vi "Measurement API.vi"(7 "Action":T1, 8 "error IO":errorcluster) -> (0 "error IO 2":errorcluster, 2 "Temps":dbl[](array[numeric]))   [LabVIEW 2019]
uses:
  <vilib>/ULx/Create Channel.llb/ULx Create Channel (AI-Temperature).vi
  <vilib>/Utility/error.llb/DialogType.ctl
  <vilib>/ULx/Read.llb/ULx Read (Analog 1D DBL NChan 1Samp).vi
  <vilib>/Utility/file.llb/Read From Spreadsheet File (DBL).vi
  Measurement Action.ctl
panel:
  out "Mtr Brg Offsets":dbl[](array[numeric]) format="%0.3f"
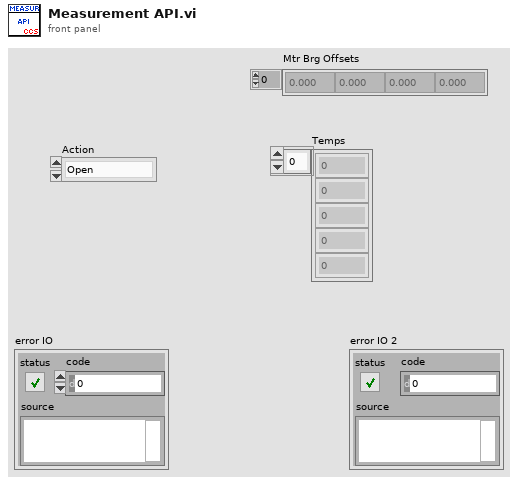
[diagram p1: front panel]
types:
  T1 = typedef "Measurement Action.ctl" = enum16{"Open", "Read Bearing Temps", "Read Motor Temps", "Close"}
  T2 = typedef "DialogType.ctl" = u16
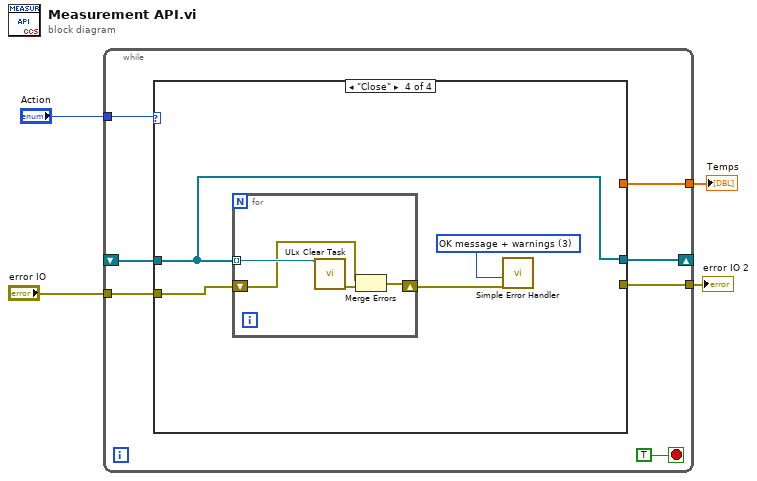
[diagram p0: block diagram]
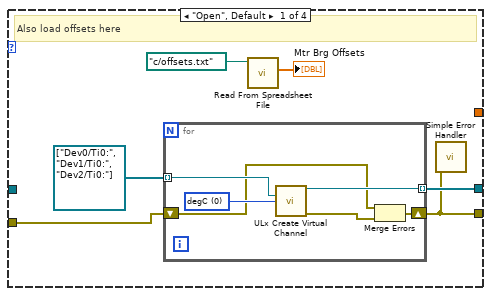
[diagram p2: hidden frame]
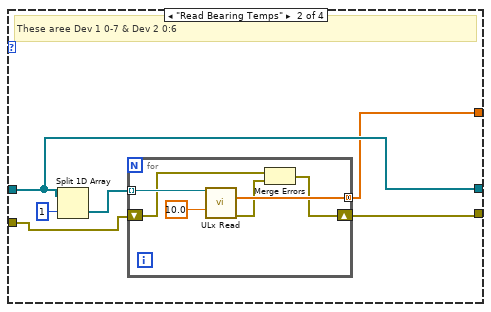
[diagram p3: hidden frame]
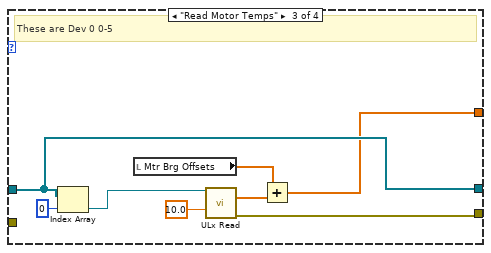
[diagram p4: hidden frame]
diagram:
  n1 = while {
    tunnel: "Action" -> [w10]
    tunnel: "error IO" -> [w8]
    tunnel: [w7] -> w2
    shift-right: [w9] -> _
    shift-left: _ -> [w6]
    tunnel: [w5] -> w1
    stop <- TRUE stop-if-true
    n2 = case shown="\"Close\"" w10 {
      tunnel: [w16 w25 w41 w45] -> w9
      tunnel: w8 -> [w15 w27 _ w44]
      tunnel: [w14 w26 w39 _] -> w7
      tunnel: w6 -> [_ w25 w41 w45]
      tunnel: [_ w24 w36 _] -> w5
      frame "Open", Default {
        # "Also load offsets here"
        n3 = for {
          tunnel: refnum<k21>[] ["Dev0/Ti0:", "Dev1/Ti0:", "Dev2/Ti0:"] -> [w22] mode=indexing
          tunnel: [w21] -> w16 mode=indexing
          shift-right: [w19] -> w14
          shift-left: w15 -> [w18]
          w23 = 0 items=["degC", "degF", "kelvin", "raw"] ("units")
          n4 = call-poly <vilib>:"ULx Create Virtual Channel.vi"("physical channels"=w22, "units"=w23) -> ("task out"=w21:refnum<k24>, "error out"=w20:errorcluster)  [unwired: 12 in]
          n5 = Merge Errors(w18, w20) -> (w19:errorcluster)
        }
        n6 = call-poly <vilib>:"Read From Spreadsheet File.vi"("file path (dialog if empty)"=path "c:/offsets.txt") -> ("first row"=→"Mtr Brg Offsets":dbl[])  [unwired: 3 in, 7 out]
        n7 = call <vilib>:"Simple Error Handler.vi"("error in (no error)"=w14) -> ()  [unwired: 4 in, 5 out]
      }
      frame "Read Bearing Temps" {
        # "These aree Dev 1 0-7 & Dev 2 0:6"
        n8 = Split 1D Array(array=w25, index=1) -> (second subarray=w28:refnum<k24>[])  [unwired: 1 out]
        n9 = for {
          tunnel: w28 -> [w34] mode=indexing
          tunnel: [w33] -> w24 mode=concatenating
          shift-right: [w30] -> w26
          shift-left: w27 -> [w32]
          n10 = call-poly <vilib>:"ULx Read.vi"("task in"=w34, "timeout"=10.0) -> ("data"=w33:dbl[], "error out"=w31:errorcluster)  [unwired: 11 in, 1 out]
          n11 = Merge Errors(w32, w31) -> (w30:errorcluster)
        }
      }
      frame "Read Motor Temps" {
        # "These are Dev 0 0-5"
        n12 = Index Array(array=w41, index=0) -> (element=w42:refnum<k24>)
        n13 = local read "Mtr Brg Offsets"() -> (w38:dbl[])
        n14 = call-poly <vilib>:"ULx Read.vi"("task in"=w42, "timeout"=10.0) -> ("data"=w37:dbl[], "error out"=w39:errorcluster)  [unwired: 11 in, 1 out]
        n15 = Add(x=w38, y=w37) -> (x+y=w36:dbl[])
      }
      frame "Close" {
        w47 = T2 3 items=["no dialog", "OK message", "continue or stop message", "OK message + warnings", "continue/stop + warnings"] ("type of dialog (OK msg:1)")
        n16 = for {
          tunnel: w45 -> [w51] mode=indexing
          shift-right: [w48] -> w46
          shift-left: w44 -> [w49]
          n17 = call <vilib>:"ULx Clear Task.vi"("task in"=w51) -> ("error out"=w50:errorcluster)  [unwired: 14 in]
          n18 = Merge Errors(w49, w50) -> (w48:errorcluster)
        }
        n19 = call <vilib>:"Simple Error Handler.vi"("type of dialog (OK msg:1)"=w47, "error in (no error)"=w46) -> ()  [unwired: 3 in, 5 out]
      }
    }
  }
  "error IO 2" <- w2
  "Temps" <- w1
